vi "reference setup.vi"() -> (3 "reference setup out":T1={"integration time"=0.5, "rinse time"=10.0, "sample time"=10.0, "sample type"=0} {"sample type" items=["Sample Cuvet", "Sipper Cell", "No Dialog"]; "sample time" min=0.0 max=100.0 step=1.0 format="%.1f"; "rinse time" min=0.0 max=100.0 step=1.0 format="%.1f"; "integration time" format="%.1f"})   [LabVIEW 2015]
uses:
  settings.ctl
panel:
  in  "ok":bool
  in  "reference setup":T1={"integration time"=0.5, "rinse time"=0.0, "sample time"=20.0, "sample type"=1} {"sample type" items=["Sample Cuvet", "Sipper Cell", "No Dialog"]; "sample time" min=0.0 max=100.0 step=1.0 format="%.1f"; "rinse time" min=0.0 max=100.0 step=1.0 format="%.1f"; "integration time" format="%.1f"}
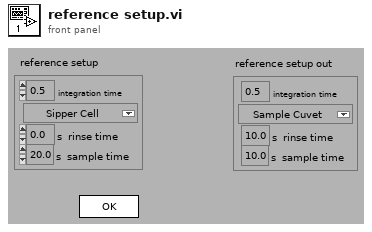
[diagram p1: front panel]
types:
  T1 = typedef "settings.ctl" = cluster{"integration time":sgl, "rinse time":dbl[unit], "sample time":dbl[unit], "sample type":u16}
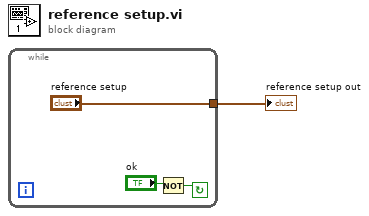
[diagram p0: block diagram]
diagram:
  n1 = while {
    tunnel: ["reference setup"] -> w1
    stop <- w3 continue-if-true
    n2 = Not(x="ok") -> (.not. x?=w3:bool)
  }
  "reference setup out" <- w1
